vi "Write to Temp File Single Channel.vi"(6 "Append to file?":bool, 8 "error in (no error)":errorcluster, 10 "Dev1 Zero Values":dbl[](array[numeric]), 11 "Waveform Array":waveform(dbl)[][](array[waveform])) -> (0 "error out":errorcluster, 2 "Fx and Fy":dbl[](array[numeric]), 3 "Zeroed Array":waveform(dbl)[][](array[waveform]))   [LabVIEW 2017]
uses:
  <vilib>/Waveform/WDTFileIO.llb/ Write Waveforms to File (1D).vi
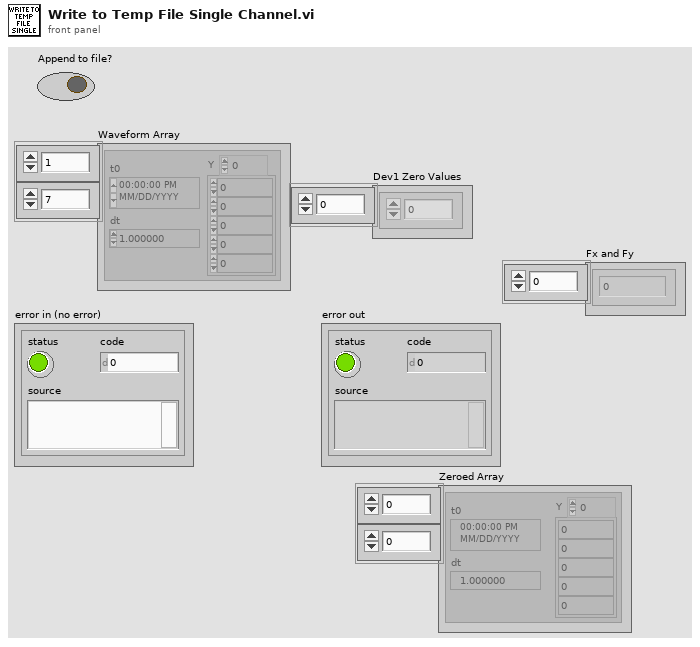
[diagram p1: front panel]
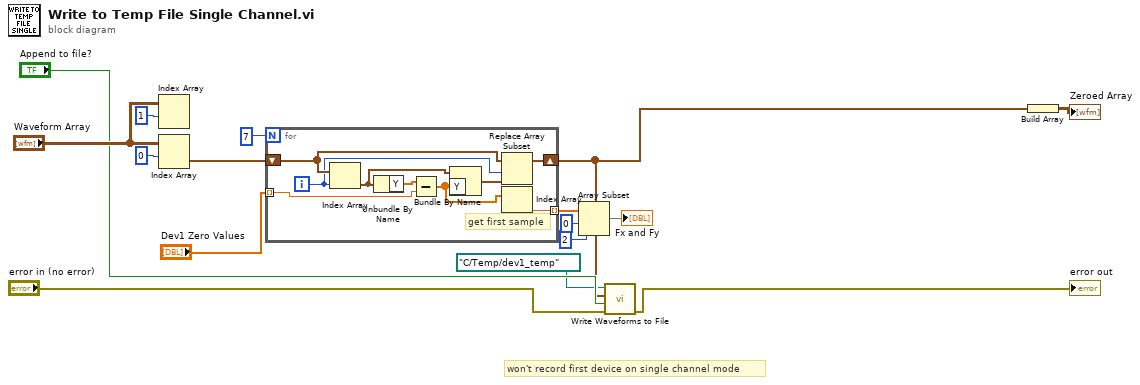
[diagram p0: block diagram]
diagram:
  # "won't record first device on single channel mode"
  n1 = Index Array(array="Waveform Array", index (row)=1) -> ()  [unwired: 1 in, 1 out]
  n2 = Index Array(array="Waveform Array", index (row)=0) -> (element=w8:waveform(dbl)[])  [unwired: 1 in]
  n3 = for {
    N: 7 -> [_]
    tunnel: "Dev1 Zero Values" -> [w24] mode=indexing
    shift-right: [w19] -> w13
    shift-left: w8 -> [w22]
    tunnel: [w17] -> w4 mode=indexing
    i -> [w21]
    # "get first sample"
    n4 = Index Array(array=w22, index=w21) -> (element=w23:waveform(dbl))
    n5 = Unbundle By Name(w23) -> ("Y"=w25:dbl[])
    n6 = Subtract(x=w25, y=w24) -> (x-y=w18:dbl[])
    n7 = Bundle By Name(cluster=w23, "Y"=w18) -> (w20:waveform(dbl))
    n8 = Replace Array Subset(array=w22, new element=w20, index=w21) -> (w19:waveform(dbl)[])
    n9 = Index Array(array=w18) -> (element=w17:dbl)  [unwired: 1 in]
  }
  n10 = Array Subset(array=w4, index=0, length=2) -> (→"Fx and Fy":dbl[])
  n11 = call-poly <vilib>:"Write Waveforms to File.vi"("error in (no error)"="error in (no error)", "append to file? (new file:F)"="Append to file?", "waveform array"=w13, "file path (dialog if empty)"=path "C:/Temp/dev1_temp") -> ("error out"=→"error out":errorcluster)  [unwired: 6 in, 1 out]
  n12 = Build Array(w13) -> (→"Zeroed Array":waveform(dbl)[][])
